vi "Populate Zip File.vi"(8 "error in (no error)":errorcluster, 10 "Source":path=path "examples/Synchronization", 11 "zip file in":i64) -> (0 "error out":errorcluster, 3 "zip file out":i64)   [LabVIEW 2020]
doc: "This VI will zip up a source directory into a Zip file."
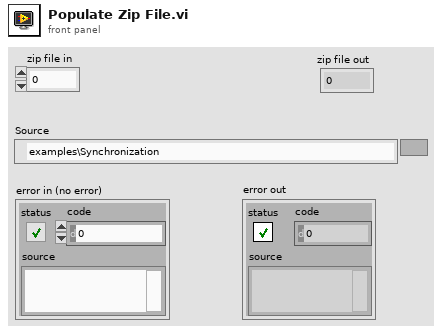
[diagram p1: front panel]
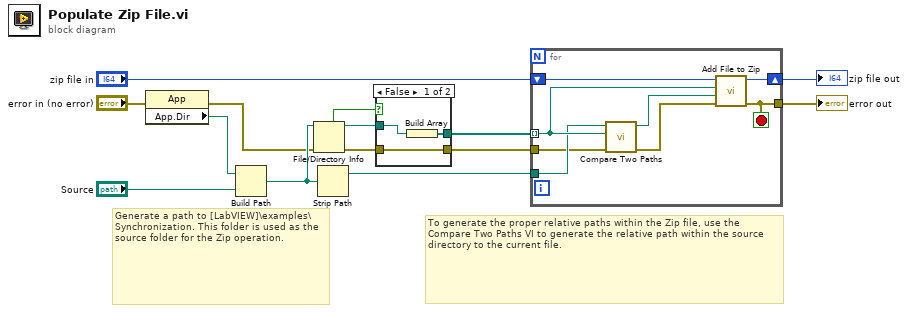
[diagram p0: block diagram]
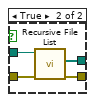
[diagram p2: hidden frame]
diagram:
  # "Generate a path to [LabVIEW]\\examples\\Synchronization. This folder is used as the source folder for the Zip operation."
  # "To generate the proper relative paths within the Zip file, use the Compare Two Paths VI to generate the relative path within the source directory to the current file."
  n1 = property class="App"(error in="error in (no error)") -> (error out=w1:errorcluster, "App.Dir"=w12:path)  [unwired: 1 in, 1 out]
  n2 = Build Path(base path=w12, name or relative path="Source") -> (appended path=w6:path)
  n3 = File/Directory Info(path=w6, error in=w1) -> (path out=w5:path, directory=w4:bool, error out=w7:errorcluster)  [unwired: 4 out]
  n4 = Strip Path(path=w6) -> (stripped path=w3:path)  [unwired: 1 out]
  n5 = case shown="False" w4 {
    tunnel: [w15 w21] -> w13
    tunnel: [w17 w20] -> w10
    tunnel: w7 -> [w17 w19]
    tunnel: w5 -> [w16 w18]
    frame False {
      n6 = Build Array(w16) -> (w15:path[])
    }
    frame True {
      n7 = call <vilib>:"Recursive File List.vi"("error in (no error)"=w19, "Folder Path"=w18) -> ("error out"=w20:errorcluster, "All Files in Dir"=w21:path[])  [unwired: 5 in, 3 out]
    }
  }
  n8 = for {
    tunnel: w13 -> [w26] mode=indexing
    tunnel: w10 -> [w23]
    tunnel: [w27] -> w8
    shift-right: [w28] -> w14
    shift-left: "zip file in" -> [w29]
    tunnel: w3 -> [w25]
    stop <- w27 stop-if-true
    n9 = call <vilib>:"Compare Two Paths.vi"("error in (no error)"=w23, "Path 2"=w26, "Path 1"=w25) -> ("error out"=w22:errorcluster, "Relative Path from 1 to 2"=w24:path)  [unwired: 5 in, 2 out]
    n10 = call <vilib>:"Add File to Zip.vi"("error in (no error)"=w22, "destination path in zip"=w24, "source file path"=w26, "zip file in"=w29) -> ("error out"=w27:errorcluster, "zip file out"=w28:i64)  [unwired: 6 out]
  }
  "error out" <- w8
  "zip file out" <- w14
